vi "Drive Handler.vi"(10 "JoystickDevRef":T1) -> ()   [LabVIEW 2019]
uses:
  <vilib>/Rock Robotics/WPI/Joystick/WPI_JoystickDevRef.ctl
  <vilib>/Rock Robotics/WPI/Joystick/WPI_JoystickDeviceEnum.ctl
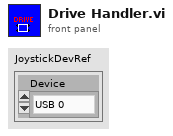
[diagram p1: front panel]
types:
  T1 = typedef "WPI_JoystickDevRef.ctl" = cluster{"Device":T2}
  T2 = typedef "WPI_JoystickDeviceEnum.ctl" = enum16{"USB 0", "USB 1", "USB 2", "USB 3", "USB 4", "USB 5"}
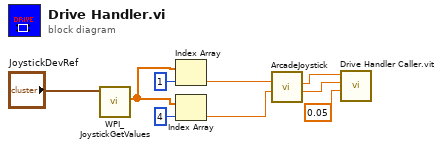
[diagram p0: block diagram]
diagram:
  n1 = call <vilib>:"WPI_JoystickGetValues.vi"("JoystickDevRef"="JoystickDevRef") -> ("Axes"=w4:dbl[])  [unwired: 6 in, 4 out]
  n2 = Index Array(array=w4, index=1) -> (element=w7:dbl)
  n3 = Index Array(array=w4, index=4) -> (element=w6:dbl)
  n4 = call "ArcadeJoystick.vi"("Y axis value"=w6, "X axis value"=w7) -> ("Right Motor Value"=w2:dbl, "Left Motor Value"=w3:dbl)  [unwired: 8 in]
  n5 = call "Drive Handler Caller.vit"("Deadband Value"=0.05, "Right Setpoint"=w2, "Setpoint"=w3) -> ()  [unwired: 8 in, 1 out]
